vi "UI Main.vi"() -> ()   [LabVIEW 2018]
uses:
  State.ctl
  UI DATA.ctl
  Classes/Config_Read/Config_Read_BML.lvclass
  SPI/Config Read SPI/Config_Read_SPI.lvclass
  Classes/BML_DigiPattern_Generator/DigiPattern_Generator.lvclass
  Classes/BML_Frame_Write_Opcode/BML_Frame_Write_Opcode.lvclass
  C:/Users/ziwang/Desktop/BML_Pattern_Gen_Refactor/Classes/BML_Frame_Root/BML_Frame_Root.lvclass
  Classes/BML_Frame_RW/BML_Frame_RW.lvclass
  Classes/BML_Frame_Read/BML_Frame_Read.lvclass
  SPI/SPI Frame Write/SPI_Frame_Write.lvclass
  C:/Users/ziwang/Desktop/BML_Pattern_Gen_Refactor/SPI/SPI Frame Root/SPI_Frame_Root.lvclass
  SPI/SPI Frame WR/SPI_Frame_WR.lvclass
  SPI/SPI Frame Read Data/SPI_Frame_Read_Data.lvclass
panel:
  in  "stop":bool
  out "error out":errorcluster
  in  "error in (no error)":errorcluster
  in  "Tab Control":enum32{"BeamLink", "SPI"}(tab)=enum."SPI"
  in  "Gen All File":bool
  in  "Gen Single File":bool
  in  "PinMap":path
  in  "Config Path":path
  in  "Timeset between frms":u32=40
  in  "# Timeset for Rd Wait":u8=1
  in  "Timeset between frms SPI":u32=40
  in  "PinMap SPI":path=path "C:/Users/8135/Desktop/BML_Pattern_Gen/BeamLink_Pattern_Gen/BML_Pattern_Gen_Refactor/SPI/Fornax_V200_B11.pinmap"
  in  "Config Path SPI":path=path "C:/Users/8135/Desktop/BML_Pattern_Gen/BeamLink_Pattern_Gen/BML_Pattern_Gen_Refactor/SPI/ConfigFiles/Fornax_ART_V201_B11_TX_reg_XCH_FIN_RX.csv"
  in  "Gen One File SPI":bool
  in  "Gen all File SPI":bool
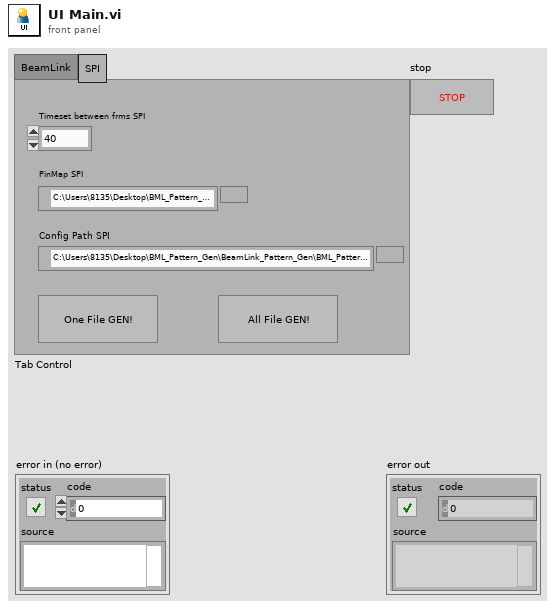
[diagram p1: front panel]
types:
  T1 = typedef "UI DATA.ctl" = cluster{"Config_Read_BML.lvclass":refnum<class "Config_Read_BML.lvclass">, "Config_Read_SPI.lvclass":refnum<class "Config_Read_SPI.lvclass">, "DigiPattern_Generator.lvclass":refnum<class "DigiPattern_Generator.lvclass">, "PinMap":path, "Config BML":path, "PinMap SPI":path, "Config  SPI":path}
  T2 = typedef "State.ctl" = enum16{"Init", "Wait for CMD", "Gen BML Pattern_ALL", "Gen BML Pattern", "Gen SPI Pattern_ALL", "Gen SPI Pattern", "Error", "End"}
  T3 = typedef "Config_Read_BML.lvclass/Frame_Data.ctl" = cluster{"Pattern_Name":string, "Operation Mode":T4, "BurstLength":T5, "FSN":u8, "Start_Addr":u16, "Data":u8[], "R/W?":T6, "Opcode":string[], "ChipID":u8, "num of wait cycle of read":i8}
  T4 = typedef "Config_Read_BML.lvclass/OperationMode.ctl" = enum8{"Normal", "ImmeEffect", "InitSlaveID", "LoadData"}
  T5 = typedef "Config_Read_BML.lvclass/BurstLength.ctl" = enum8{"0", "2", "3", "4", "5", "8", "16", "32"}
  T6 = typedef "Config_Read_BML.lvclass/RW_Option.ctl" = enum16{"Read", "Write", "R/W"}
  T7 = typedef "Config_Read_SPI.lvclass/SPI_FRM_Config.ctl" = cluster{"Pattern Name":string, "Data":u16, "Addr":u16, "R/W?":T6, "Opcode":string[], "SPI_Mode":T8}
  T8 = typedef "Config_Read_SPI.lvclass/SPI_Mode.ctl" = enum16{"SPI_3W", "SPI_4W"}
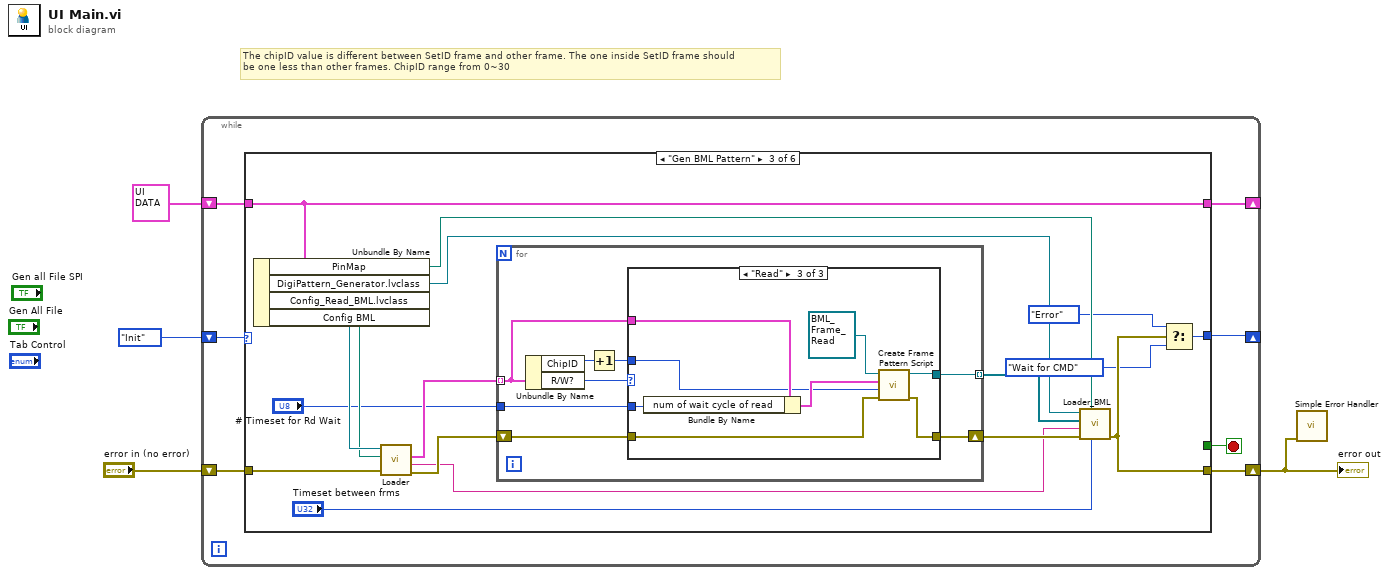
[diagram p0: block diagram]
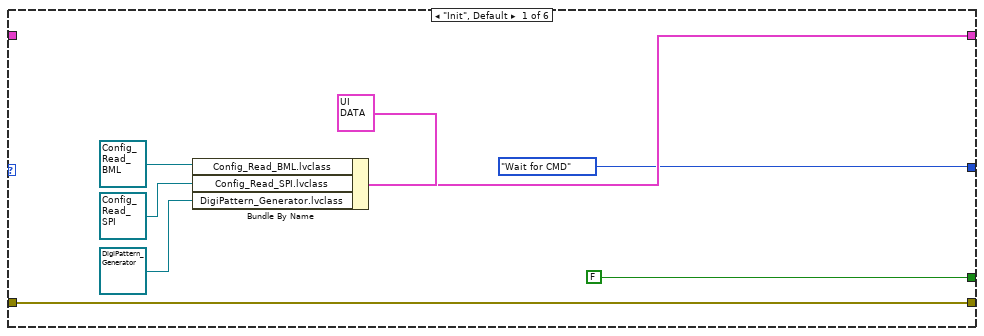
[diagram p2: hidden frame]
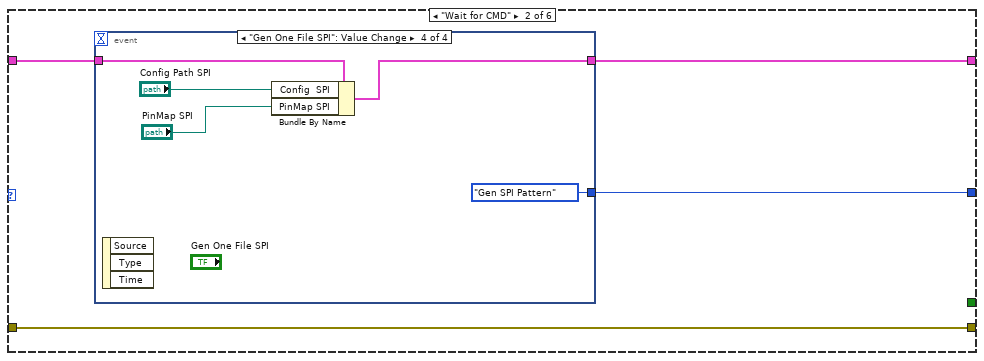
[diagram p3: hidden frame]
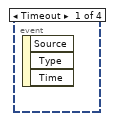
[diagram p4: hidden frame]
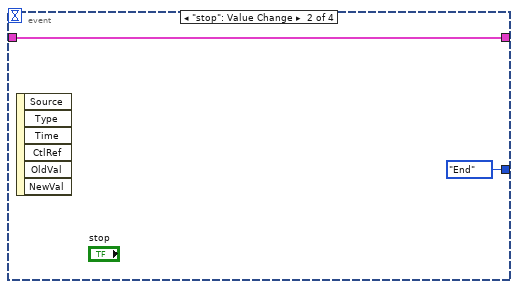
[diagram p5: hidden frame]
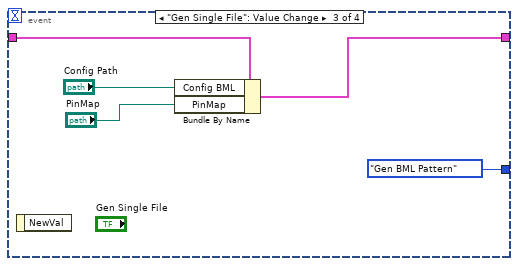
[diagram p6: hidden frame]
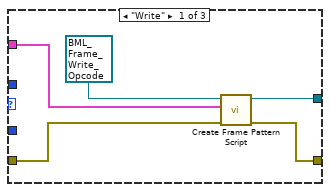
[diagram p7: hidden frame]
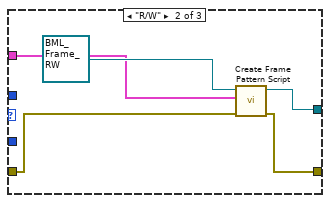
[diagram p8: hidden frame]
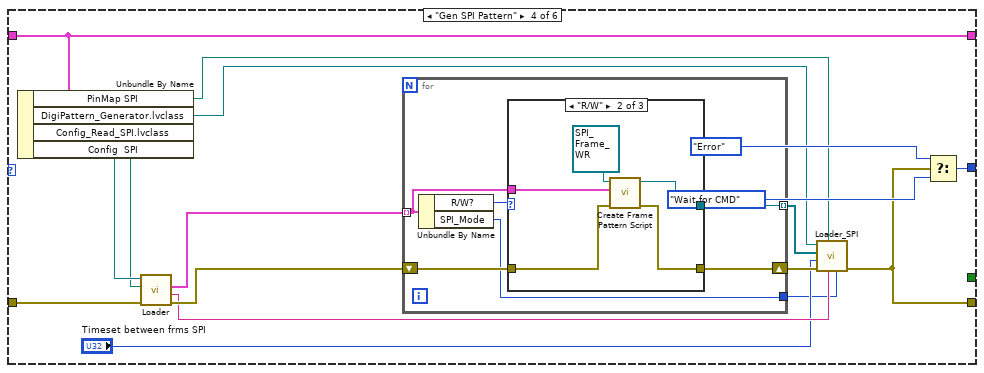
[diagram p9: hidden frame]
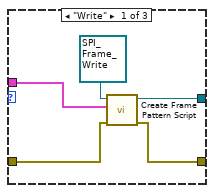
[diagram p10: hidden frame]
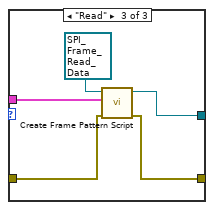
[diagram p11: hidden frame]
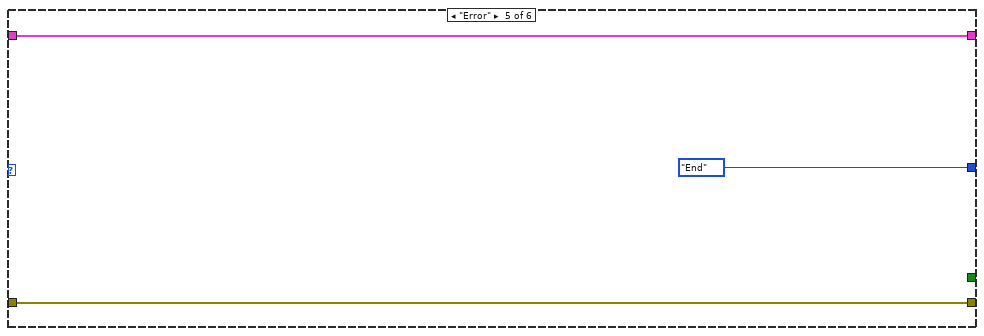
[diagram p12: hidden frame]
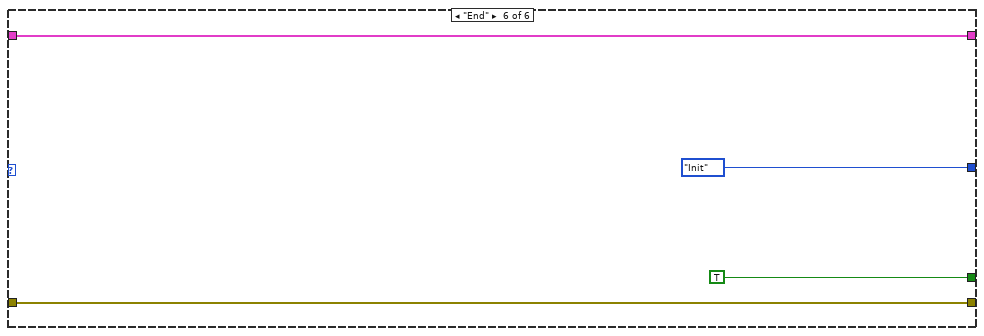
[diagram p13: hidden frame]
diagram:
  # "The chipID value is different between SetID frame and other frame. The one inside SetID frame should \nbe one less than other frames. ChipID range from 0~30"
  n1 = while {
    shift-right: [w5] -> _
    shift-left: State."Init" -> [w11]
    shift-right: [w6] -> w1
    shift-left: "error in (no error)" -> [w10]
    shift-right: [w8] -> _
    shift-left: T1 {"Config_Read_BML.lvclass"=refnum, "Config_Read_SPI.lvclass"=refnum, "DigiPattern_Generator.lvclass"=refnum, "PinMap"=path "", "Config BML"=path "", "PinMap SPI"=path "", "Config  SPI"=path ""} ("UI DATA") -> [w7]
    stop <- w9 stop-if-true
    n2 = case shown="\"Gen BML Pattern\"" w11 {
      tunnel: w10 -> [w13 w21 w52 w90 w119 w121]
      tunnel: [FALSE _ _ _ _ TRUE] -> w9
      tunnel: [w14 w22 w41 w95 w117 w120] -> w8
      tunnel: w7 -> [_ w23 w41 w95 w117 w120]
      tunnel: [w13 w21 w40 w80 w119 w121] -> w6
      tunnel: [State."Wait for CMD" w20 w39 w94 State."End" State."Init"] -> w5
      frame "Init", Default {
        n3 = Bundle By Name(cluster=T1 {"Config_Read_BML.lvclass"=refnum, "Config_Read_SPI.lvclass"=refnum, "DigiPattern_Generator.lvclass"=refnum, "PinMap"=path "", "Config BML"=path "", "PinMap SPI"=path "", "Config  SPI"=path ""} ("UI DATA"), "Config_Read_BML.lvclass"=refnum<class "Config_Read_BML.lvclass"> refnum, "Config_Read_SPI.lvclass"=refnum<class "Config_Read_SPI.lvclass"> refnum, "DigiPattern_Generator.lvclass"=refnum<class "DigiPattern_Generator.lvclass"> refnum) -> (w14:T1)
      }
      frame "Wait for CMD" {
        n4 = event shown="[3] \"Gen One File SPI\": Value Change" {
          selector: _ -> [_ _ _ _]
          dyn-events: _ -> [_ _ _ _]
          timeout: _ -> [_ _ _ _]
          tunnel: w23 -> [_ w25 w30 w34]
          tunnel: [_ w25 w27 w31] -> w22
          tunnel: [_ State."End" State."Gen BML Pattern" State."Gen SPI Pattern"] -> w20
          event Timeout {
            n5 = event-data() -> ()  [unwired: 1 in, 3 out]
          }
          event "stop": Value Change {
            n6 = event-data() -> ()  [unwired: 1 in, 6 out]
          }
          event "Gen Single File": Value Change {
            n7 = event-data() -> ()  [unwired: 1 in, 1 out]
            n8 = Bundle By Name(cluster=w30, "Config BML"="Config Path", "PinMap"="PinMap") -> (w27:T1)
          }
          event "Gen One File SPI": Value Change {
            n9 = event-data() -> ()  [unwired: 1 in, 3 out]
            n10 = Bundle By Name(cluster=w34, "Config  SPI"="Config Path SPI", "PinMap SPI"="PinMap SPI") -> (w31:T1)
          }
        }
      }
      frame "Gen BML Pattern" {
        n11 = Unbundle By Name(w41) -> ("PinMap"=w44:path, "DigiPattern_Generator.lvclass"=w45:refnum<class "DigiPattern_Generator.lvclass">, "Config_Read_BML.lvclass"=w51:refnum<class "Config_Read_BML.lvclass">, "Config BML"=w50:path)
        n12 = call "Loader.vi"("error in (no error)"=w52, "Path"=w50, "Config_Read.lvclass"=w51) -> ("error out"=w49:errorcluster, "Pattern_Name"=w42:string, "FRM_Data_Array"=w48:T3[])  [unwired: 5 in, 1 out]
        n13 = for {
          tunnel: w48 -> [w58] mode=indexing
          shift-right: [w57] -> w46
          shift-left: w49 -> [w59]
          tunnel: [w56] -> w47 mode=indexing
          tunnel: "# Timeset for Rd Wait" -> [w55]
          n14 = Unbundle By Name(w58) -> ("ChipID"=w54:u8, "R/W?"=w60:T6)
          n15 = Increment(x=w54) -> (x+1=w53:u8)
          n16 = case shown="\"Read\"" w60 {
            tunnel: w59 -> [w64 w68 w76]
            tunnel: w58 -> [w65 w69 w74]
            tunnel: [w63 w66 w77] -> w56
            tunnel: [w62 w67 w75] -> w57
            tunnel: w55 -> [_ _ w72]
            tunnel: w53 -> [_ _ w71]
            frame "Write" {
              n17 = call-dynamic "Create Frame Pattern Script.vi"("error in (no error)"=w64, "Frame_Data"=w65, "BML_Frame_Write_Opcode in"=refnum<class "BML_Frame_Write_Opcode.lvclass"> refnum ("BML_Frame_Write_Opcode.lvclass")) -> ("error out"=w62:errorcluster, "BML_Frame_Write_Opcode out"=w63:refnum<class "BML_Frame_Write_Opcode.lvclass">)  [unwired: 7 in]
            }
            frame "R/W" {
              n18 = call-dynamic "Create Frame Pattern Script.vi"("error in (no error)"=w68, "Frame_Data"=w69, "BML_Frame_RW in"=refnum<class "BML_Frame_RW.lvclass"> refnum ("BML_Frame_RW.lvclass")) -> ("error out"=w67:errorcluster, "BML_Frame_RW out"=w66:refnum<class "BML_Frame_RW.lvclass">)  [unwired: 7 in]
            }
            frame "Read" {
              n19 = Bundle By Name(cluster=w74, "num of wait cycle of read"=w72) -> (w73:T3)
              n20 = call-dynamic "Create Frame Pattern Script.vi"("error in (no error)"=w76, "ChipID"=w71, "Frame_Data"=w73, "BML_Frame_Read in"=refnum<class "BML_Frame_Read.lvclass"> refnum ("BML_Frame_Read.lvclass")) -> ("error out"=w75:errorcluster, "BML_Frame_Read out"=w77:refnum<class "BML_Frame_Read.lvclass">)  [unwired: 6 in]
            }
          }
        }
        n21 = call "Loader_BML.vi"("Timeset between frms"="Timeset between frms", "PinMap"=w44, "error in (no error)"=w46, "Pattern Name"=w42, "BML Frame Array"=w47, "BML_DigiPattern_Generator.lvclass"=w45) -> ("error out"=w40:errorcluster)  [unwired: 4 in, 1 out]
        n22 = Select(t=State."Error", s=w40, f=State."Wait for CMD") -> (s? t:f=w39:T2)
      }
      frame "Gen SPI Pattern" {
        n23 = Unbundle By Name(w95) -> ("PinMap SPI"=w82:path, "DigiPattern_Generator.lvclass"=w84:refnum<class "DigiPattern_Generator.lvclass">, "Config_Read_SPI.lvclass"=w91:refnum<class "Config_Read_SPI.lvclass">, "Config  SPI"=w89:path)
        n24 = call "Loader.vi"("error in (no error)"=w90, "Path"=w89, "Config_Read_SPI.lvclass"=w91) -> ("error out"=w88:errorcluster, "Pattern_Name"=w85:string, "SPI_FRM_Array"=w87:T7[])  [unwired: 5 in, 1 out]
        n25 = for {
          shift-right: [w99] -> w86
          shift-left: w88 -> [w100]
          tunnel: w87 -> [w97] mode=indexing
          tunnel: [w98] -> w83 mode=indexing
          tunnel: [w96] -> w79
          n26 = Unbundle By Name(w97) -> ("R/W?"=w101:T6, "SPI_Mode"=w96:T8)
          n27 = case shown="\"R/W\"" w101 {
            tunnel: w100 -> [w104 w111 w116]
            tunnel: [w103 w110 w115] -> w99
            tunnel: [w105 w107 w112] -> w98
            tunnel: w97 -> [w102 w108 w114]
            frame "Write" {
              n28 = call-dynamic "Create Frame Pattern Script.vi"("error in (no error)"=w104, "SPI_FRM_Config"=w102, "SPI_Frame_Write in"=refnum<class "SPI_Frame_Write.lvclass"> refnum ("SPI_Frame_Write.lvclass")) -> ("error out"=w103:errorcluster, "SPI_Frame_Write out"=w105:refnum<class "SPI_Frame_Write.lvclass">)  [unwired: 7 in]
            }
            frame "R/W" {
              n29 = call-dynamic "Create Frame Pattern Script.vi"("error in (no error)"=w111, "SPI_FRM_Config"=w108, "SPI_Frame_WR in"=refnum<class "SPI_Frame_WR.lvclass"> refnum ("SPI_Frame_WR.lvclass")) -> ("error out"=w110:errorcluster, "SPI_Frame_WR out"=w107:refnum<class "SPI_Frame_WR.lvclass">)  [unwired: 7 in]
            }
            frame "Read" {
              n30 = call-dynamic "Create Frame Pattern Script.vi"("error in (no error)"=w116, "SPI_FRM_Config"=w114, "SPI_Frame_Read_Data in"=refnum<class "SPI_Frame_Read_Data.lvclass"> refnum ("SPI_Frame_Read_Data.lvclass")) -> ("error out"=w115:errorcluster, "SPI_Frame_Read_Data out"=w112:refnum<class "SPI_Frame_Read_Data.lvclass">)  [unwired: 7 in]
            }
          }
        }
        n31 = call "Loader_SPI.vi"("SPI_Mode"=w79, "Pattern Name"=w85, "PinMap"=w82, "error in (no error)"=w86, "Timeset between frms"="Timeset between frms SPI", "SPI Frame Array"=w83, "DigiPattern_Generator.lvclass"=w84) -> ("error out"=w80:errorcluster)  [unwired: 3 in, 1 out]
        n32 = Select(t=State."Error", s=w80, f=State."Wait for CMD") -> (s? t:f=w94:T2)
      }
      frame "Error" {
      }
      frame "End" {
      }
    }
  }
  "error out" <- w1
  n33 = call <vilib>:"Simple Error Handler.vi"("error in (no error)"=w1) -> ()  [unwired: 4 in, 5 out]
